vi "Remove Image Outliers.vi"(8 "error in (no error)":errorcluster, 9 "Percentile (0-100, Default: ignore)":dbl min=0.0 max=100.0, 10 "Delta (Default: ignore)":sgl=inf, 11 "Refnum in":T1) -> (0 "error out":errorcluster, 3 "Refnum out":T1)   [LabVIEW 2021]
uses:
  <vilib>/vision/Image Controls.llb/IMAQ Image.ctl
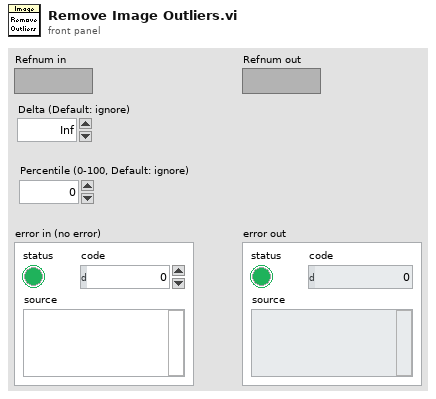
[diagram p1: front panel]
types:
  T1 = typedef "IMAQ Image.ctl" = refnum<image>
  T2 = typedef "Image Type" = u32
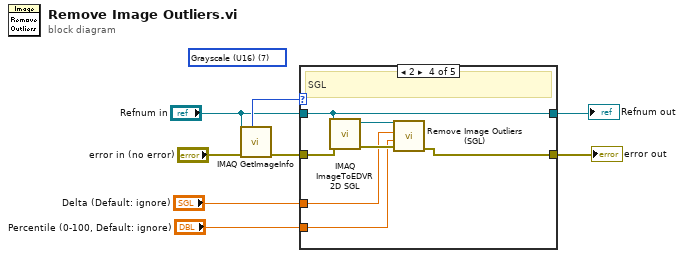
[diagram p0: block diagram]
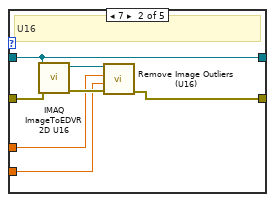
[diagram p3: hidden frame]
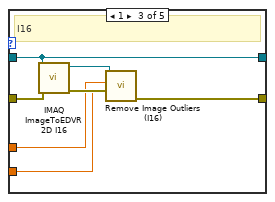
[diagram p4: hidden frame]
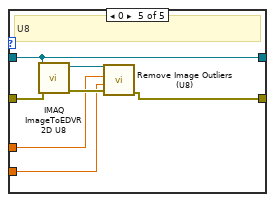
[diagram p5: hidden frame]
diagram:
  (unwired) T2 7 items=["Grayscale (U8)", "Grayscale (I16)", "Grayscale (SGL)", "Complex (CSG)", "RGB (U32)", "HSL (U32)", "RGB (U64)", "Grayscale (U16)"] ("Image Type")
  n1 = call "IMAQ GetImageInfo"("error in (no error)"="error in (no error)", "Image"="Refnum in") -> ("error out"=w4:errorcluster, "Image Type"=w7:T2)  [unwired: 2 in, 6 out]
  n2 = case shown="2" w7 {
    tunnel: "Refnum in" -> [w10 w17 w24 w31 w38]
    tunnel: [w10 w17 w24 w31 w38] -> w5
    tunnel: w4 -> [w9 w16 w23 w30 w37]
    tunnel: [w9 w13 w20 w27 w34] -> w3
    tunnel: "Delta (Default: ignore)" -> [_ w12 w19 w26 w33]
    tunnel: "Percentile (0-100, Default: ignore)" -> [_ w11 w18 w25 w32]
    frame 3, Default {
      # "unsupported"
    }
    frame 7 {
      # "U16"
      n3 = call <vilib>:"IMAQ ImageToEDVR 2D U16.vi"("error out"=w16, "Image"=w17) -> ("error out"=w14:errorcluster, "EDVR 2D U16"=w15:refnum<data-value>)  [unwired: 7 in, 1 out]
      n4 = call "Remove Image Outliers (U16).vi"("error in (no error)"=w14, "Percentile (0-100, Default: ignore)"=w11, "Delta (Default: ignore)"=w12, "Data Value Reference in"=w15) -> ("error out"=w13:errorcluster)  [unwired: 7 in]
    }
    frame 1 {
      # "I16"
      n5 = call <vilib>:"IMAQ ImageToEDVR 2D I16.vi"("error in (no error)"=w23, "Image"=w24) -> ("error out"=w21:errorcluster, "EDVR 2D I16"=w22:refnum<data-value>)  [unwired: 7 in, 1 out]
      n6 = call "Remove Image Outliers (I16).vi"("error in (no error)"=w21, "Percentile (0-100, Default: ignore)"=w18, "Delta (Default: ignore)"=w19, "Data Value Reference in"=w22) -> ("error out"=w20:errorcluster)  [unwired: 7 in]
    }
    frame 2 {
      # "SGL"
      n7 = call <vilib>:"IMAQ ImageToEDVR 2D SGL.vi"("error in (no error)"=w30, "Image"=w31) -> ("error out"=w28:errorcluster, "EDVR 2D SGL"=w29:refnum<data-value>)  [unwired: 7 in, 1 out]
      n8 = call "Remove Image Outliers (SGL).vi"("error in (no error)"=w28, "Percentile (0-100, Default: ignore)"=w25, "Delta (Default: ignore)"=w26, "Data Value Reference in"=w29) -> ("error out"=w27:errorcluster)  [unwired: 7 in]
    }
    frame 0 {
      # "U8"
      n9 = call <vilib>:"IMAQ ImageToEDVR 2D U8.vi"("error in (no error)"=w37, "Image"=w38) -> ("error out"=w35:errorcluster, "EDVR 2D U8"=w36:refnum<data-value>)  [unwired: 7 in, 1 out]
      n10 = call "Remove Image Outliers (U8).vi"("error in (no error)"=w35, "Percentile (0-100, Default: ignore)"=w32, "Delta (Default: ignore)"=w33, "Data Value Reference in"=w36) -> ("error out"=w34:errorcluster)  [unwired: 7 in]
    }
  }
  "Refnum out" <- w5
  "error out" <- w3
